vi "PPR_SIM_ENCODER_ALLOC.vi"() -> (3 "Encoder Index":T1)   [LabVIEW 2019]
uses:
  <vilib>/Rock Robotics/SystemInterfaces/Encoder/FPGA_EncoderIdx.ctl
  PPR_SIM_SIM_Globals.vi
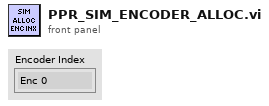
[diagram p1: front panel]
types:
  T1 = typedef "FPGA_EncoderIdx.ctl" = enum8{"Enc 0", "Enc 1", "Enc 2", "Enc 3", "Enc 4", "Enc 5", "Enc 6", "Enc 7", "Invalid"}
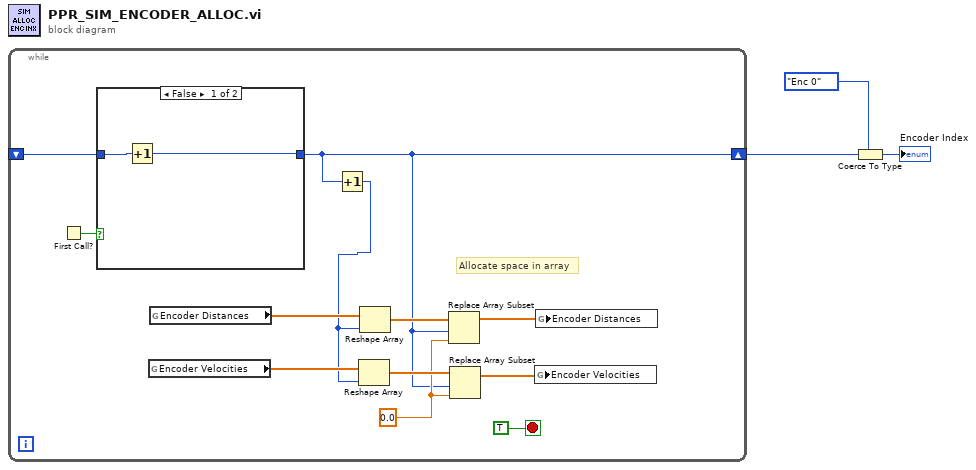
[diagram p0: block diagram]
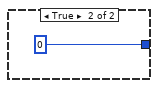
[diagram p2: hidden frame]
diagram:
  n1 = while {
    shift-right: [w4] -> w2
    shift-left: _ -> [w13]
    stop <- TRUE stop-if-true
    w7 = 0.0 ("new element/subarray")
    # "Allocate space in array"
    n2 = First Call?() -> (First Call?: T/F=w14:bool)
    n3 = case shown="False" w14 {
      tunnel: [w16 0] -> w4
      tunnel: w13 -> [w17 _]
      frame False {
        n4 = Increment(x=w17) -> (x+1=w16:i32)
      }
      frame True {
      }
    }
    n5 = global read "PPR_SIM_SIM_Globals.vi" "Encoder Velocities"() -> (w11:dbl[])
    n6 = global read "PPR_SIM_SIM_Globals.vi" "Encoder Distances"() -> (w12:dbl[])
    n7 = Increment(x=w4) -> (x+1=w8:i32)
    n8 = Reshape Array(w11, w8) -> (w9:dbl[])
    n9 = Reshape Array(w12, w8) -> (w10:dbl[])
    n10 = Replace Array Subset(array=w10, new element=w7, index=w4) -> (w6:dbl[])
    n11 = Replace Array Subset(array=w9, new element=w7, index=w4) -> (w5:dbl[])
    n12 = global write "PPR_SIM_SIM_Globals.vi" "Encoder Velocities"(w5) -> ()
    n13 = global write "PPR_SIM_SIM_Globals.vi" "Encoder Distances"(w6) -> ()
  }
  n14 = Coerce To Type(0:w2, 1:FPGA_EncoderIdx."Enc 0" ("EncoderIndex")) -> (2:→"Encoder Index":T1)
